vi "YTO_check_lock_Naoj.vi"(5 "Cartridge band":u32 max=10 step=1, 7 "Slave Node in":cluster{"Address":i16, "Serial Number":i8[]}={"Address"=19, "Serial Number"=[16, 71, 55, 76, 1, 8, 0, -15]} {"Serial Number" format="%.0x"; "Address" format="%.0x"}, 8 "error IO":errorcluster, 11 "ObjHandle in":u32) -> (0 "error":errorcluster, 1 "Lock":bool, 3 "ObjHandle out":u32)   [LabVIEW 2017]
panel:
  # "Node Address"
  # "Serial Number"
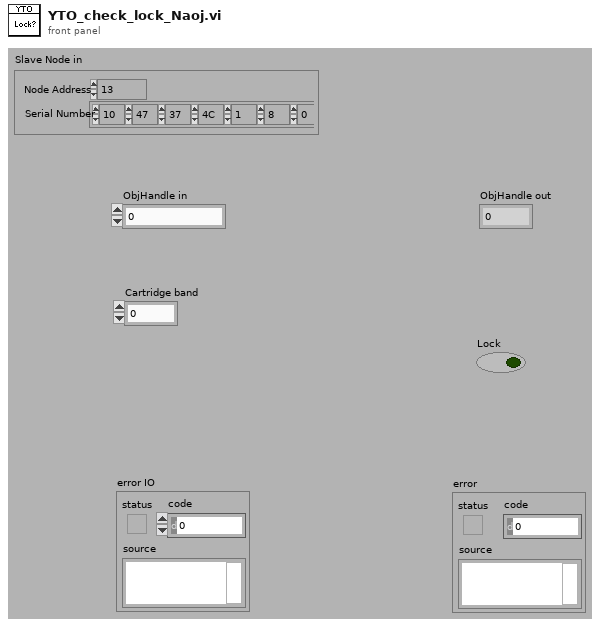
[diagram p1: front panel]
types:
  T1 = cluster{"PLL_ASSY_T":sgl, "PLL_REF_TOT_P":sgl, "PLL_IF_TOT_P":sgl, "PLL_CORR_V":sgl, "PLL_LOCK_V":sgl, "PLL_5V_SUPPLY_V":sgl, "Temp_TF":bool, "PLL Ref Pwr_TF":bool, "IF Pwr_TF":bool, "PLL Corr_TF":bool, "PLL Lock V_TF":bool, "PLL Nominal_TF":bool}
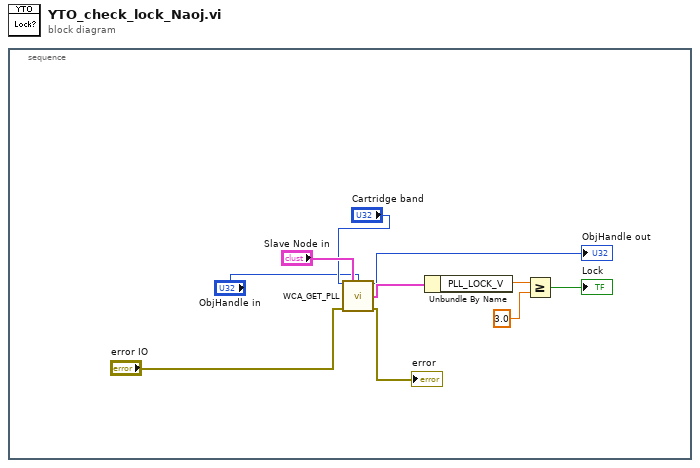
[diagram p0: block diagram]
diagram:
  n1 = stacked-sequence {
    frame #0 {
      n2 = call "WCA_GET_PLL.vi"("Cartridge Band"="Cartridge band", "Slave Node in"="Slave Node in", "ObjHandle in"="ObjHandle in", "error in (no error)"="error IO") -> ("ObjHandle out"=→"ObjHandle out":u32, "GET_PLL"=w7:T1, "error out"=→"error":errorcluster)  [unwired: 9 in]
      n3 = Unbundle By Name(w7) -> ("PLL_LOCK_V"=w8:sgl)
      n4 = Greater Or Equal?(x=w8, y=sgl 3.0) -> (x >= y?=→"Lock":bool)
    }
  }
